vi "Check.vi"(0 "BroadcastRegistry In":T3, 5 "Broadcast":string, 7 "SourceCSM":string, 11 "TargetCSM":string) -> (4 "BroadcastRegistry Out":T3, 6 "Response Message Info":T1[](array[typedef]))   [LabVIEW 2017, in "Communicable State Machine.lvlib"]
doc: "### Check.vi\n\n-- <b>Controls</b> --\n- <b>BroadcastRegistry in</b>:\n- <b>Status</b>:\n- <b>Source</b>:\n- <b>Target</b>:\n\n-- <b>Indicators</b> --\n- <b>BroadcastRegistry out</b>:\n- <b>Response Message Info</b>:"
uses:
  Communicable State Machine.lvlib
  BroadcastRegistry.ctl
  BroadcastRegistry-Value.ctl
  AdvanceAPI/CSM - Broadcast Message Type.ctl
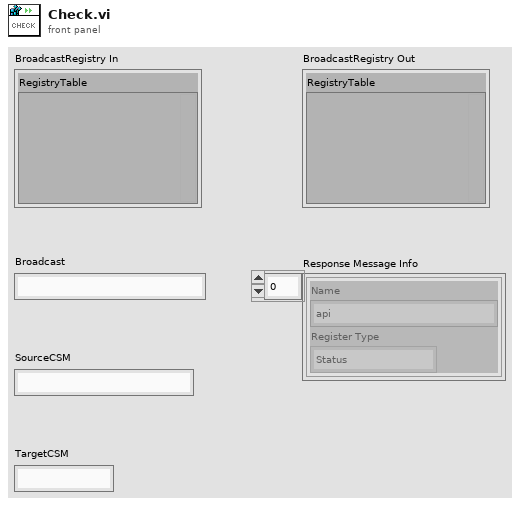
[diagram p1: front panel]
types:
  T1 = typedef "Communicable State Machine.lvlib/BroadcastRegistry-Value.ctl" = cluster{"Name":string, "Register Type":T2}
  T2 = typedef "Communicable State Machine.lvlib/CSM - Broadcast Message Type.ctl" = enum16{"<Null>", "Status", "Interrupt"}
  T3 = typedef "Communicable State Machine.lvlib/BroadcastRegistry.ctl" = cluster{"RegistryTable":variant}
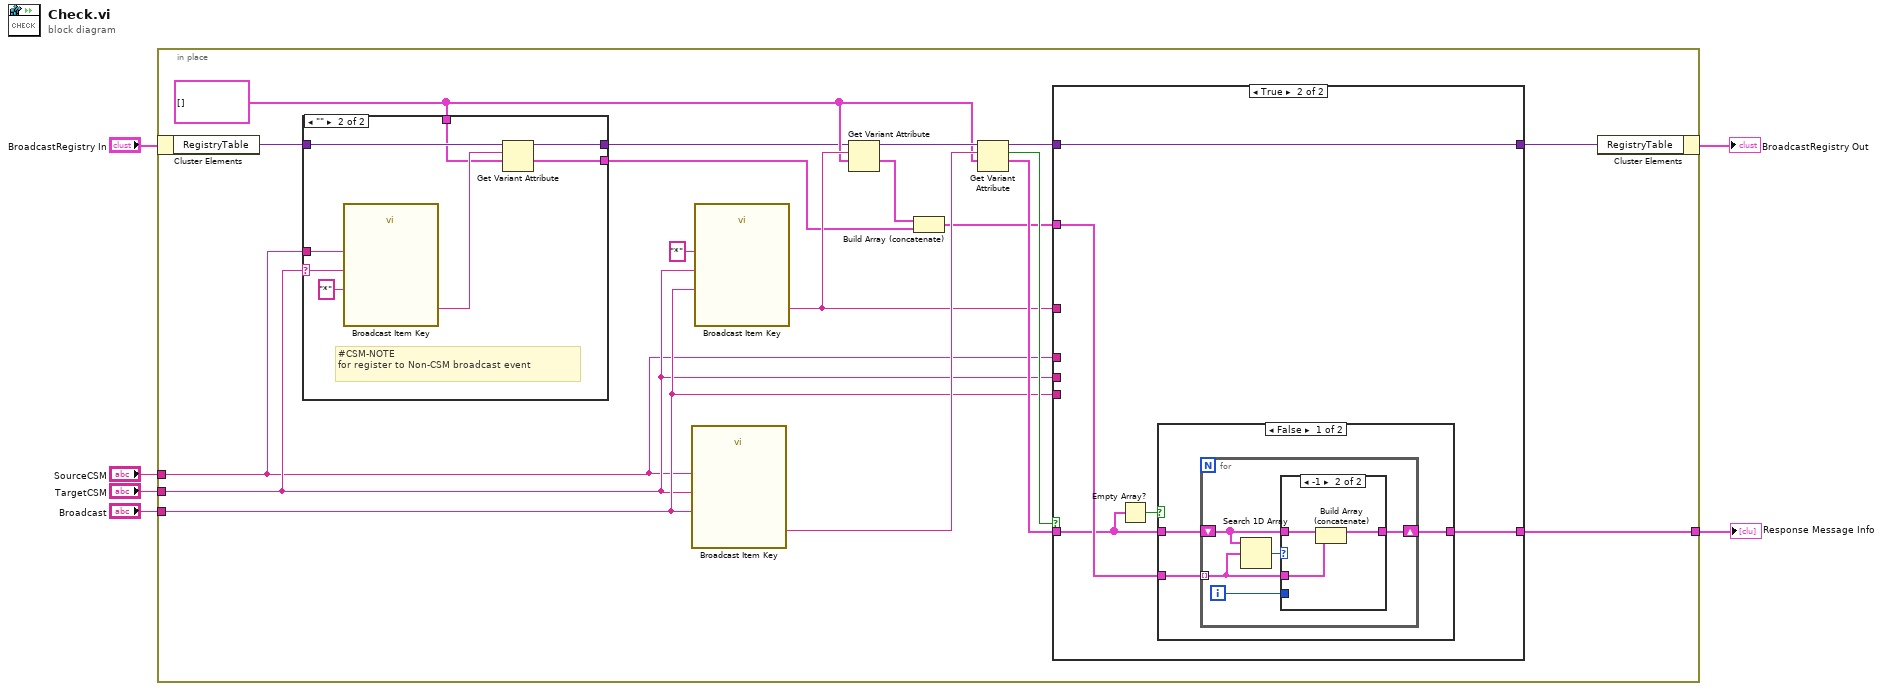
[diagram p0: block diagram]
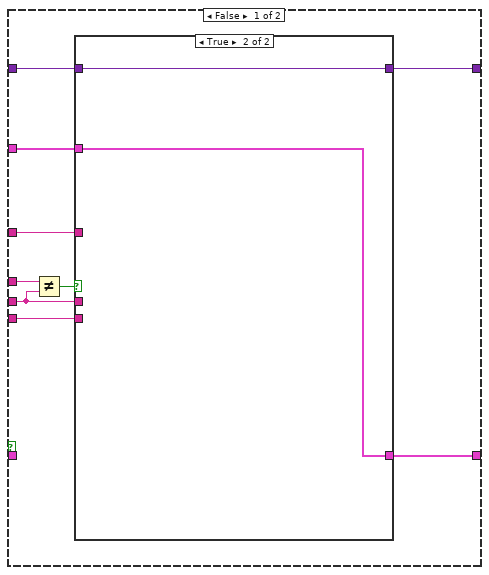
[diagram p3: hidden frame]
diagram:
  n1 = in-place {
    in-place-border: "Broadcast" -> [w17]
    in-place-border: "TargetCSM" -> [w13]
    in-place-border: "SourceCSM" -> [w12]
    in-place-border: [w20] -> w1
    w10 = T1[] [] ("Response Message Info")
    n2 = in-place-cluster #1("BroadcastRegistry In") -> ("RegistryTable"=w11:variant)
    n3 = case shown="\"\"" w13 {
      selector: w13 -> [_ w33]
      tunnel: w12 -> [_ w32]
      tunnel: w11 -> [w25 w30]
      tunnel: w10 -> [_ w28]
      tunnel: [w25 w27] -> w9
      tunnel: [_ w26] -> w7
      frame Default {
      }
      frame "" {
        # "#CSM-NOTE\nfor register to Non-CSM broadcast event"
        n4 = call "Broadcast Item Key.vi"("Status"="*", "Target"=w33, "Source"=w32) -> ("Key"=w29:string)  [unwired: 2 in]
        n5 = Get Variant Attribute(Variant=w30, name=w29, default value (empty Variant)=w28) -> (duplicate Variant=w27:variant, value=w26:T1[])  [unwired: 1 in, 2 out]
      }
    }
    n6 = call "Broadcast Item Key.vi"("Status"=w17, "Target"=w13, "Source"=w12) -> ("Key"=w24:string)  [unwired: 2 in]
    n7 = call "Broadcast Item Key.vi"("Status"=w17, "Target"=w13, "Source"="*") -> ("Key"=w15:string)  [unwired: 2 in]
    n8 = Get Variant Attribute(Variant=w9, name=w15, default value (empty Variant)=w10) -> (duplicate Variant=w16:variant, value=w14:T1[])  [unwired: 1 in, 2 out]
    n9 = Build Array (concatenate)(w14, w7) -> (w8:T1[])
    n10 = Get Variant Attribute(Variant=w16, name=w24, default value (empty Variant)=w10) -> (duplicate Variant=w23:variant, found=w22:bool, value=w19:T1[])  [unwired: 1 in, 1 out]
    n11 = case shown="True" w22 {
      tunnel: w17 -> [w42 _]
      tunnel: w13 -> [w37 _]
      tunnel: w23 -> [w41 w50]
      tunnel: [w40 w50] -> w21
      tunnel: w19 -> [_ w47]
      tunnel: [w39 w48] -> w20
      tunnel: w12 -> [w38 _]
      tunnel: w15 -> [w35 _]
      tunnel: w8 -> [w34 w49]
      frame False {
        n12 = Not Equal?(x=w38, y=w37) -> (x != y?=w36:bool)
        n13 = case shown="True" w36 {
          tunnel: w42 -> [_ _]
          tunnel: w37 -> [_ _]
          tunnel: w41 -> [w43 w45]
          tunnel: [w43 w45] -> w40
          tunnel: [_ w44] -> w39
          tunnel: w35 -> [_ _]
          tunnel: w34 -> [_ w44]
          frame False {
          }
          frame True {
          }
        }
      }
      frame True {
        n14 = Empty Array?(array=w47) -> (empty?=w46:bool)
        n15 = case shown="False" w46 {
          tunnel: w49 -> [w53 _]
          tunnel: [w52 w63] -> w48
          tunnel: w47 -> [w51 w63]
          frame False {
            n16 = for {
              tunnel: w53 -> [w57] mode=indexing
              shift-right: [w56] -> w52
              shift-left: w51 -> [w55]
              i -> [w54]
              n17 = Search 1D Array(1D array=w55, element=w57) -> (index of element=w58:i32)  [unwired: 1 in]
              n18 = case shown="-1" w58 {
                tunnel: w57 -> [_ w62]
                tunnel: [w59 w60] -> w56
                tunnel: w55 -> [w59 w61]
                tunnel: w54 -> [_ _]
                frame Default {
                }
                frame -1 {
                  n19 = Build Array (concatenate)(w61, w62) -> (w60:T1[])
                }
              }
            }
          }
          frame True {
          }
        }
      }
    }
    n20 = in-place-cluster #1("RegistryTable"=w21) -> (→"BroadcastRegistry Out":T3)
  }
  "Response Message Info" <- w1
